vi "Impulsator_reg.vi"(7 "Initialise":bool, 9 "proportional gain (Kc)":dbl=0.1 format="%.3f", 10 "PV":dbl format="%#.1g", 11 "upper limit":dbl=100.0 format="%#_13g") -> (3 "Y":bool)   [LabVIEW 2019, in "Userlib.lvlib"]
uses:
  Userlib.lvlib
  Reg/control.lvlib
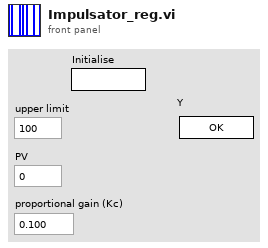
[diagram p1: front panel]
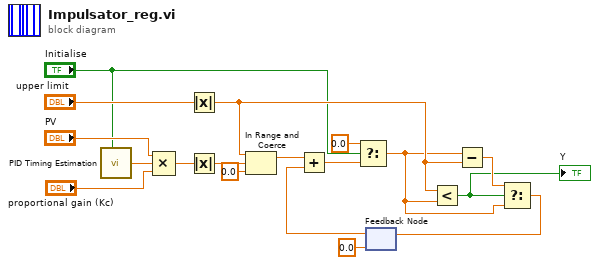
[diagram p0: block diagram]
diagram:
  n1 = call "PID Timing Estimation.vi"("R"="Initialise") -> ("dt (s) out"=w7:dbl)  [unwired: 8 in]
  n2 = Compound Arithmetic op=MULTIPLY("PV", w7, "proportional gain (Kc)") -> (w4:dbl)
  n3 = Absolute Value(x="upper limit") -> (abs(x)=w10:dbl)
  n4 = Absolute Value(x=w4) -> (abs(x)=w9:dbl)
  n5 = In Range and Coerce(upper limit=w10, x=w9, lower limit=0.0) -> (coerced(x)=w3:dbl)  [unwired: 1 out]
  n6 = feedback #1(0.0) -> (w18:dbl)
  n7 = Add(x=w3, y=w18) -> (x+y=w2:dbl)
  n8 = Select(t=0.0, s="Initialise", f=w2) -> (s? t:f=w1:dbl)
  n9 = Less?(x=w10, y=w1) -> (x < y?=w12:bool)
  "Y" <- w12
  n10 = Subtract(x=w1, y=w10) -> (x-y=w14:dbl)
  n11 = Select(t=w14, s=w12, f=w1) -> (s? t:f=w13:dbl)
  n12 = feedback-in #1(w13) -> ()
